vi "get_driver_info.vi"(2 "error in (no error)":errorcluster caption="错误输入（无错误）", 3 "StepMotor输入":refnum<class "StepMotor.lvclass">) -> (0 "error out":errorcluster caption="错误输出", 1 "driver info":T1)   [LabVIEW 2016, in "MotionControl.lvlib" / "StepMotor.lvclass"]
uses:
  <userlib>/MotionControl/StepMotor/StepMotor.lvclass
  <userlib>/MotionControl/StepMotor/DriverInfo.ctl
  <userlib>/MotionControl/StepMotor/StepMotor.lvclass/StepMotor.ctl
  <userlib>/UISimCanFunc_wrapper/UISimCanFunc_wrapper.lvlib
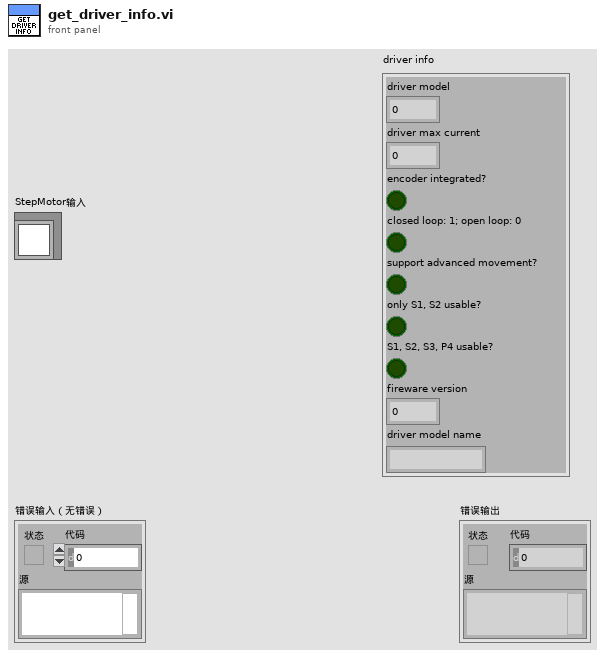
[diagram p1: front panel]
types:
  T1 = typedef "MotionControl.lvlib/StepMotor.lvclass/DriverInfo.ctl" = cluster{"driver model":u32, "driver max current":u32, "encoder integrated?":bool, "closed loop: 1; open loop: 0":bool, "support advanced movement?":bool, "only S1, S2 usable?":bool, "S1, S2, S3, P4 usable?":bool, "fireware version":u32, "driver model name":string}
  T2 = typedef "UISimCanFunc_wrapper.lvlib/MDL_INFO_OBJ.ctl" = cluster{"uiCANNodeType":u32, "uiCurrent":u32, "bIntegrationEncode":bool, "bEnCode":bool, "bMotion":bool, "b2Sensor":bool, "b4Sensor":bool, "uiFirewareVersion":u32, "szModelName":string}
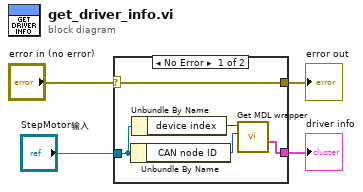
[diagram p0: block diagram]
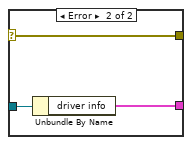
[diagram p2: hidden frame]
diagram:
  n1 = case shown="No Error" "error in (no error)" {
    selector: "error in (no error)" -> [w9 w12]
    tunnel: [w9 w12] -> w3
    tunnel: [w5 w10] -> w1
    tunnel: "StepMotor输入" -> [w8 w11]
    frame No Error {
      n2 = Unbundle By Name(w8) -> ("CAN node ID"=w6:u32)
      n3 = Unbundle By Name(w8) -> ("device index"=w7:u32)
      n4 = call <userlib>:"Get MDL wrapper.vi"("dwCanNodeId"=w6, "dwDevIndex"=w7) -> ("MDL_INFO_OBJ"=w5:T2)  [unwired: 7 in, 2 out]
    }
    frame Error {
      n5 = Unbundle By Name(w11) -> ("driver info"=w10:T1)
    }
  }
  "error out" <- w3
  "driver info" <- w1
